vi "Typhon_Software-RevE.vi"() -> ()   [LabVIEW 2020]
uses:
  <vilib>/DAQmx/write.llb/DAQmx Write (Digital 1D Bool 1Chan 1Samp).vi
  <vilib>/DAQmx/read.llb/DAQmx Read (Analog 1D DBL NChan 1Samp).vi
  <vilib>/Utility/file.llb/Write Delimited Spreadsheet (string).vi
  <vilib>/DAQmx/create/channels.llb/DAQmx Create Channel (AI-Voltage-Basic).vi
  <vilib>/DAQmx/configure/timing.llb/DAQmx Timing (Sample Clock).vi
  <vilib>/DAQmx/miscellaneous.llb/DAQmx Fill In Error Info.vi
  <vilib>/Utility/file.llb/Write Delimited Spreadsheet (DBL).vi
  <vilib>/DAQmx/create/channels.llb/DAQmx Create Channel (DO-Digital Output).vi
panel:
  out "Temp 3":dbl(graph)
  out "Temp 2":dbl(graph)
  out "Load mV":dbl(graph)
  out "time":timestamp
  in  "stop":bool
  out "Temp 1":dbl(graph)
  out "Thrust":dbl
  out "Temp 3":dbl
  out "Temp 2":dbl
  out "Temp 1":dbl
  in  "Force":path
  in  "Temperature":path
  out "E-Match":bool
  out "N2-CH4":bool
  out "N2-GOX":bool
  out "CH4  Isolation":bool
  out "CH4  Upper":bool
  out "GOX Isolation":bool
  out "GOX Upper":bool
  out "State":i32
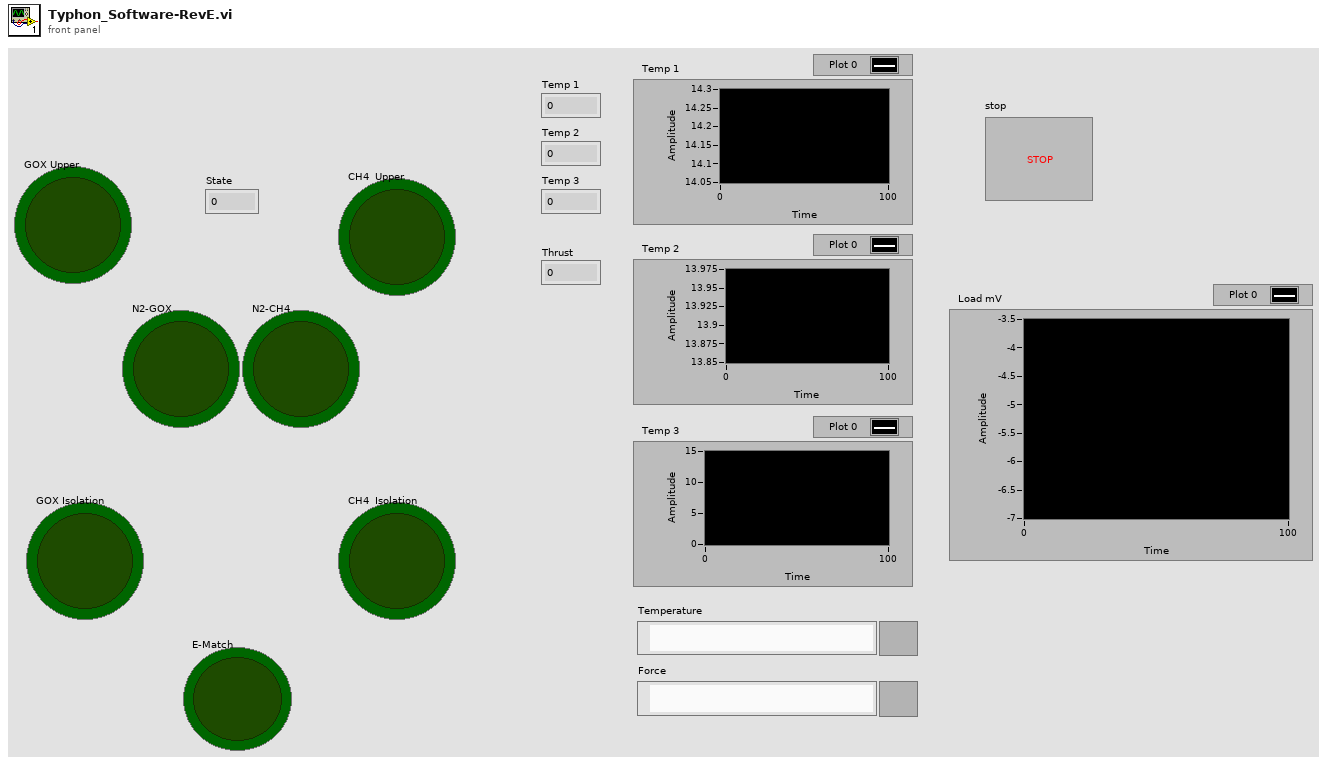
[diagram p1: front panel]
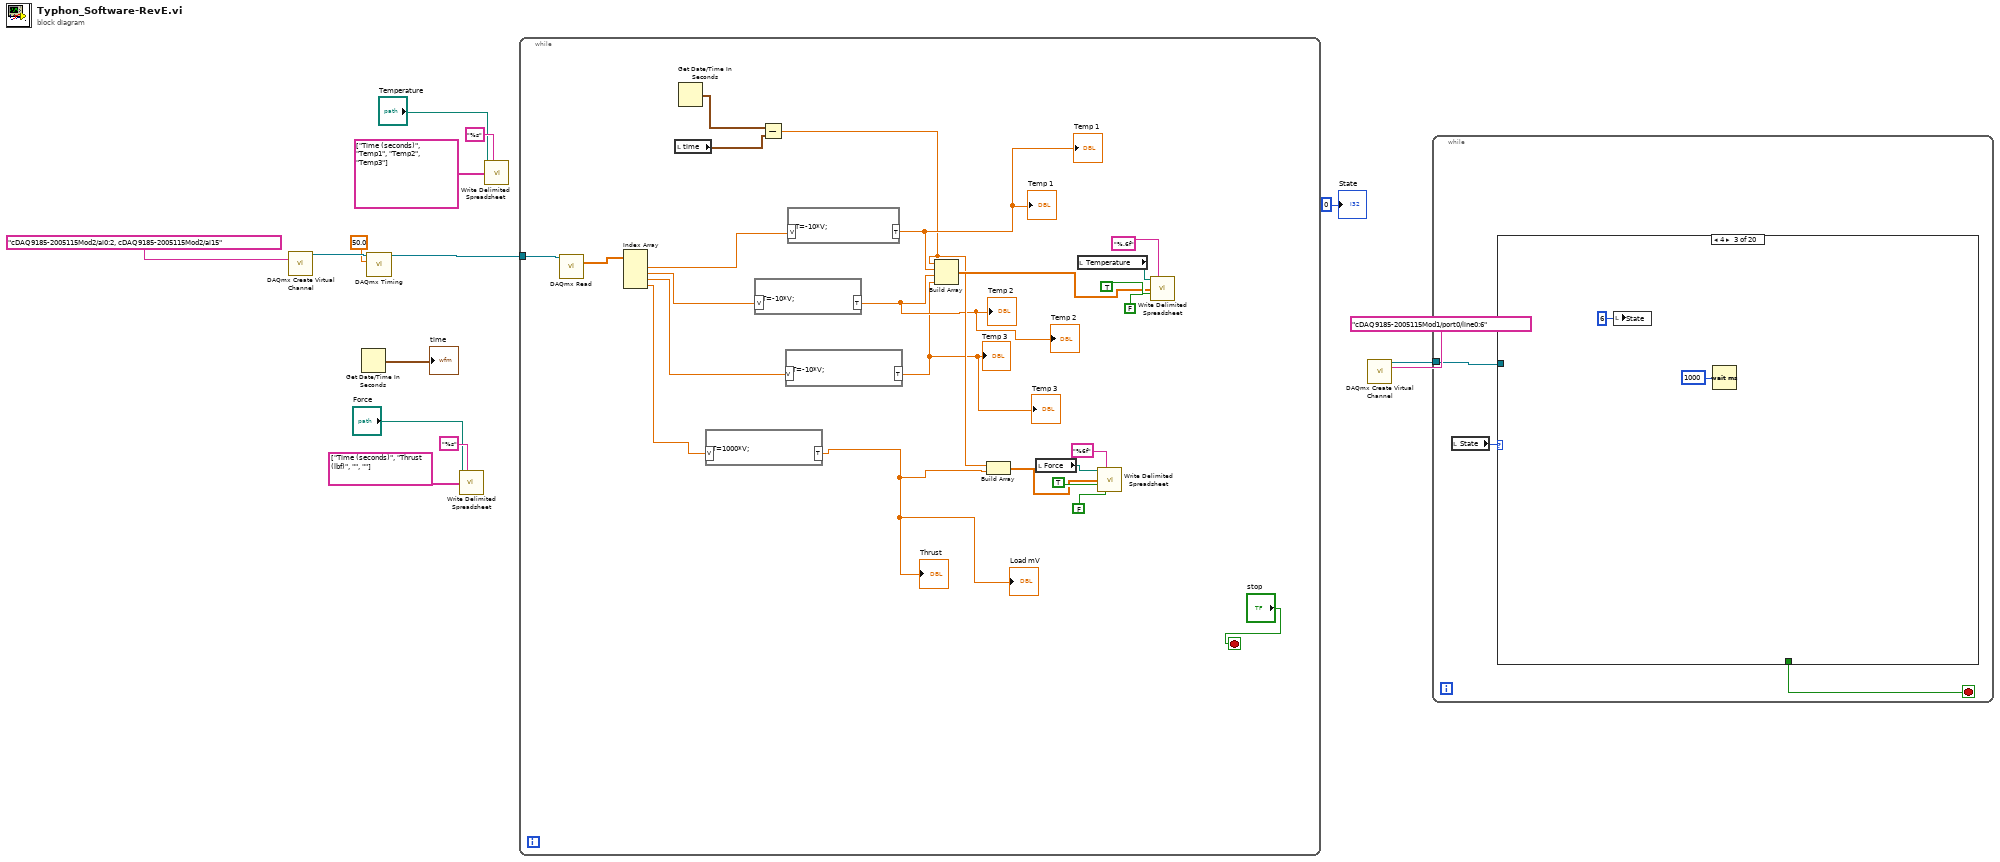
[diagram p0: block diagram]
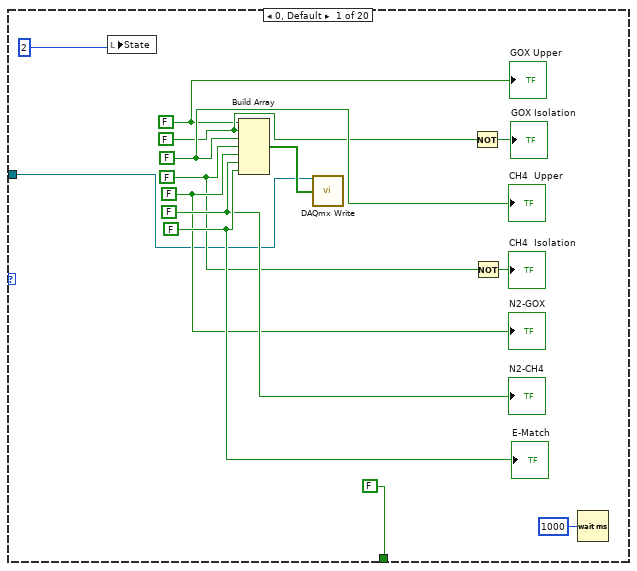
[diagram p2: hidden frame]
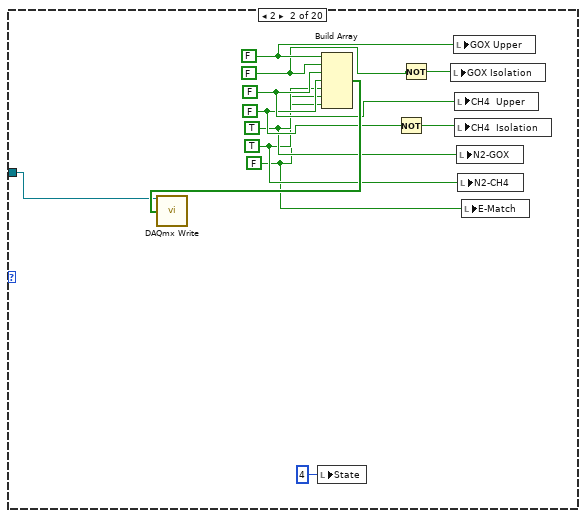
[diagram p3: hidden frame]
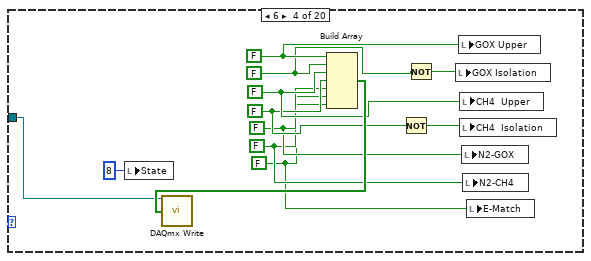
[diagram p4: hidden frame]
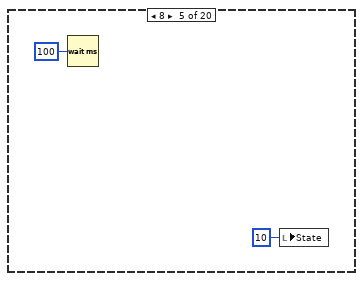
[diagram p5: hidden frame]
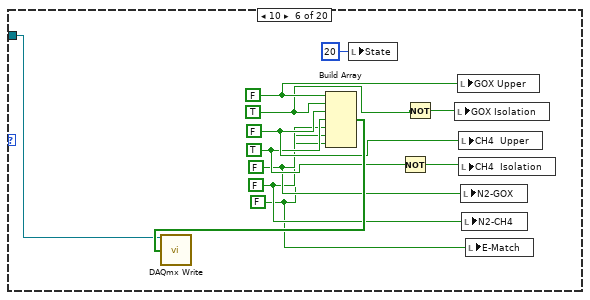
[diagram p6: hidden frame]
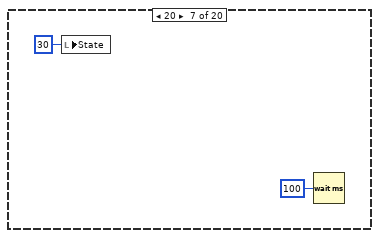
[diagram p7: hidden frame]
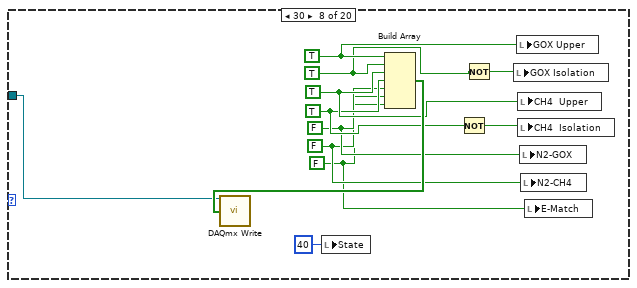
[diagram p8: hidden frame]
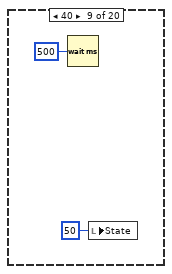
[diagram p9: hidden frame]
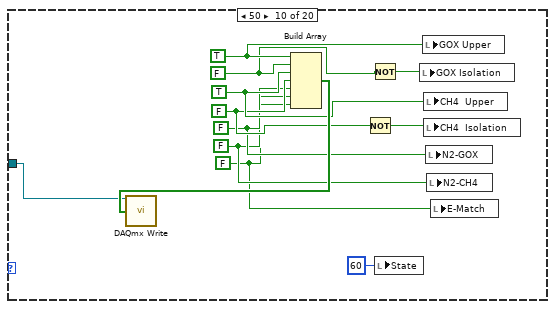
[diagram p10: hidden frame]
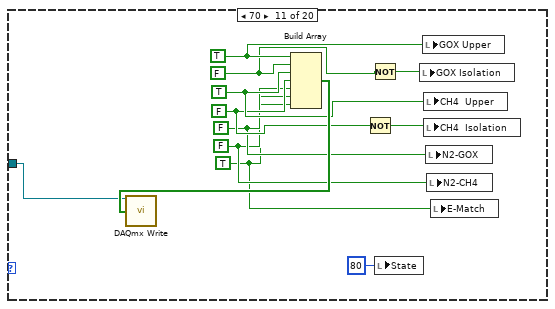
[diagram p11: hidden frame]
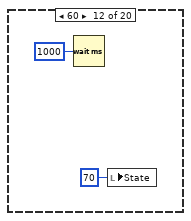
[diagram p12: hidden frame]
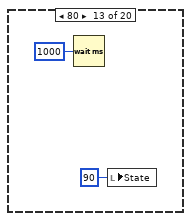
[diagram p13: hidden frame]
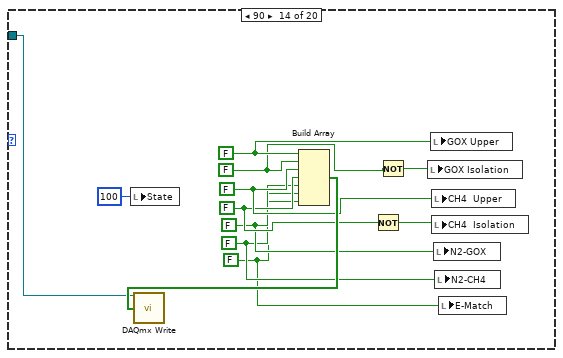
[diagram p14: hidden frame]
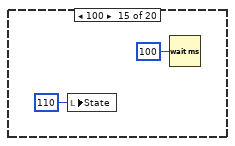
[diagram p15: hidden frame]
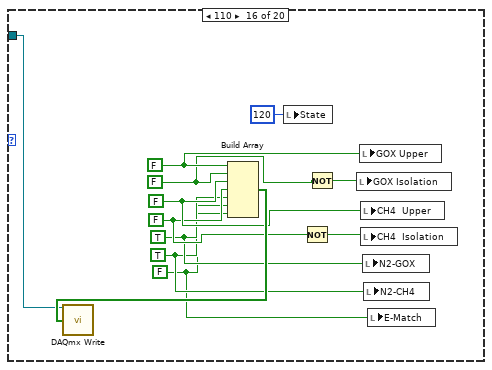
[diagram p16: hidden frame]
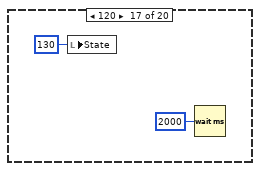
[diagram p17: hidden frame]
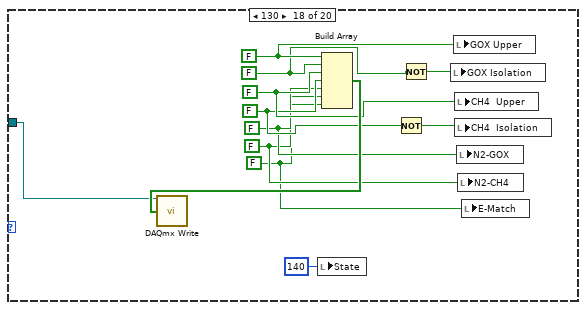
[diagram p18: hidden frame]
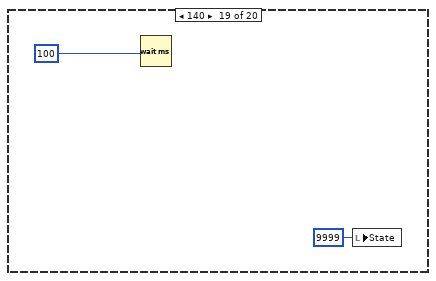
[diagram p19: hidden frame]
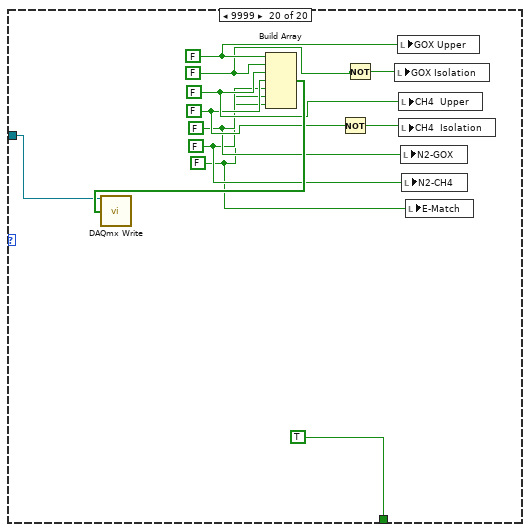
[diagram p20: hidden frame]
diagram:
  n1 = call-poly <vilib>:"DAQmx Create Virtual Channel.vi"("physical channels"=tag "cDAQ9185-2005115Mod2/ai0:2, cDAQ9185-2005115Mod2/ai15") -> ("task out"=w10:refnum<k21>)  [unwired: 13 in, 1 out]
  n2 = Get Date/Time In Seconds() -> (seconds since 1Jan1904=→"time":timestamp)
  n3 = call-poly <vilib>:"DAQmx Timing.vi"("task/channels in"=w10, "rate"=50.0) -> ("task out"=w7:refnum<k21>)  [unwired: 12 in, 1 out]
  n4 = call-poly <vilib>:"Write Delimited Spreadsheet.vi"("file path (dialog if empty)"="Force", "format (%s)"="%s" ("format (%.3f)"), "1D data"=string[] ["Time (seconds)", "Thrust (lbf)", "", ""]) -> ()  [unwired: 11 in, 2 out]
  n5 = call-poly <vilib>:"Write Delimited Spreadsheet.vi"("file path (dialog if empty)"="Temperature", "format (%s)"="%s" ("format (%.3f)"), "1D data"=string[] ["Time (seconds)", "Temp1", "Temp2", "Temp3"]) -> ()  [unwired: 11 in, 2 out]
  n6 = while {
    tunnel: w7 -> [w33]
    stop <- "stop" stop-if-true
    n7 = call-poly <vilib>:"DAQmx Read.vi"("task/channels in"=w33) -> ("data"=w34:dbl[])  [unwired: 12 in, 2 out]
    n8 = Index Array(array=w34) -> (element #1=w29:dbl, element #2=w28:dbl, element #3=w27:dbl, element #4=w18:dbl)  [unwired: 4 in]
    n9 = local read "time"() -> (w20:timestamp)
    n10 = Get Date/Time In Seconds() -> (seconds since 1Jan1904=w21:timestamp)
    n11 = formula code="T=1000*V;"("V"=w18) -> ("T"=w17:dbl)
    "Thrust" <- w17
    "Load mV" <- w17
    n12 = formula code="T=-10*V;"("V"=w28) -> ("T"=w16:dbl)
    "Temp 2" <- w16
    "Temp 2" <- w16
    n13 = Subtract(x=w21, y=w20) -> (x-y=w22:dbl)
    n14 = formula code="T=-10*V;"("V"=w27) -> ("T"=w15:dbl)
    "Temp 3" <- w15
    "Temp 3" <- w15
    n15 = formula code="T=-10*V;"("V"=w29) -> ("T"=w26:dbl)
    "Temp 1" <- w26
    "Temp 1" <- w26
    n16 = Build Array(w22, w26, w16, w15) -> (w24:dbl[])
    n17 = Build Array(w22, w17) -> (w19:dbl[])
    n18 = local read "Force"() -> (w30:path)
    n19 = local read "Temperature"() -> (w35:path)
    n20 = call-poly <vilib>:"Write Delimited Spreadsheet.vi"("file path (dialog if empty)"=w30, "format (%.3f)"="%6f", "1D data"=w19, "append to file? (new file:F)"=TRUE, "transpose? (no:F)"=FALSE) -> ()  [unwired: 9 in, 2 out]
    n21 = call-poly <vilib>:"Write Delimited Spreadsheet.vi"("file path (dialog if empty)"=w35, "format (%.3f)"="%.6f", "1D data"=w24, "append to file? (new file:F)"=TRUE, "transpose? (no:F)"=FALSE) -> ()  [unwired: 9 in, 2 out]
  }
  n22 = call-poly <vilib>:"DAQmx Create Virtual Channel.vi"("lines"=tag "cDAQ9185-2005115Mod1/port0/line0:6") -> ("task out"=w2:refnum<k21>)  [unwired: 13 in, 1 out]
  n23 = while {
    tunnel: w2 -> [w40]
    stop <- w39 stop-if-true
    n24 = local read "State"() -> (w41:i32)
    n25 = case shown="4" w41 {
      tunnel: [FALSE _ _ _ _ _ _ _ _ _ _ _ _ _ _ _ _ _ _ TRUE] -> w39
      tunnel: w40 -> [w42 w56 _ w70 _ w84 _ w98 _ w112 w124 _ _ w140 _ w154 _ w168 _ w182]
      frame 0, Default {
        w49 = FALSE ("element")
        w48 = FALSE ("element")
        w47 = FALSE ("element")
        w46 = FALSE ("element")
        w45 = FALSE ("element")
        w44 = FALSE
        w43 = FALSE
        n26 = local write "State"(2 ("State")) -> ()
        n27 = Build Array(w43, w44, w45, w46, w47, w48, w49) -> (w50:bool[])
        n28 = call-poly <vilib>:"DAQmx Write.vi"("task/channels in"=w42, "data"=w50) -> ()  [unwired: 11 in, 3 out]
        n29 = Not(x=w44) -> (.not. x?=→"GOX Isolation":bool)
        n30 = Not(x=w46) -> (.not. x?=→"CH4  Isolation":bool)
        n31 = Wait (ms)(milliseconds to wait=u32 1000) -> ()  [unwired: 1 out]
        "GOX Upper" <- w43
        "CH4  Upper" <- w45
        "N2-GOX" <- w47
        "N2-CH4" <- w48
        "E-Match" <- w49
      }
      frame 2 {
        w57 = FALSE ("element")
        w58 = TRUE ("element")
        w59 = TRUE ("element")
        w60 = FALSE ("element")
        w61 = FALSE ("element")
        w62 = FALSE
        w63 = FALSE
        n32 = local write "State"(4 ("State")) -> ()
        n33 = Build Array(w63, w62, w61, w60, w59, w58, w57) -> (w66:bool[])
        n34 = call-poly <vilib>:"DAQmx Write.vi"("task/channels in"=w56, "data"=w66) -> ()  [unwired: 11 in, 3 out]
        n35 = Not(x=w60) -> (.not. x?=w65:bool)
        n36 = Not(x=w62) -> (.not. x?=w64:bool)
        n37 = local write "GOX Isolation"(w64) -> ()
        n38 = local write "GOX Upper"(w63) -> ()
        n39 = local write "CH4  Upper"(w61) -> ()
        n40 = local write "CH4  Isolation"(w65) -> ()
        n41 = local write "N2-GOX"(w59) -> ()
        n42 = local write "N2-CH4"(w58) -> ()
        n43 = local write "E-Match"(w57) -> ()
      }
      frame 4 {
        n44 = local write "State"(6 ("State")) -> ()
        n45 = Wait (ms)(milliseconds to wait=u32 1000) -> ()  [unwired: 1 out]
      }
      frame 6 {
        w71 = FALSE ("element")
        w72 = FALSE ("element")
        w73 = FALSE ("element")
        w74 = FALSE ("element")
        w75 = FALSE ("element")
        w76 = FALSE
        w77 = FALSE
        n46 = local write "State"(8 ("State")) -> ()
        n47 = Build Array(w77, w76, w75, w74, w73, w72, w71) -> (w80:bool[])
        n48 = call-poly <vilib>:"DAQmx Write.vi"("task/channels in"=w70, "data"=w80) -> ()  [unwired: 11 in, 3 out]
        n49 = Not(x=w74) -> (.not. x?=w79:bool)
        n50 = Not(x=w76) -> (.not. x?=w78:bool)
        n51 = local write "GOX Isolation"(w78) -> ()
        n52 = local write "GOX Upper"(w77) -> ()
        n53 = local write "CH4  Upper"(w75) -> ()
        n54 = local write "CH4  Isolation"(w79) -> ()
        n55 = local write "N2-GOX"(w73) -> ()
        n56 = local write "N2-CH4"(w72) -> ()
        n57 = local write "E-Match"(w71) -> ()
      }
      frame 8 {
        n58 = Wait (ms)(milliseconds to wait=u32 100) -> ()  [unwired: 1 out]
        n59 = local write "State"(10 ("State")) -> ()
      }
      frame 10 {
        w85 = FALSE ("element")
        w86 = FALSE ("element")
        w87 = FALSE ("element")
        w88 = TRUE ("element")
        w89 = FALSE ("element")
        w90 = TRUE
        w91 = FALSE
        n60 = Build Array(w91, w90, w89, w88, w87, w86, w85) -> (w94:bool[])
        n61 = call-poly <vilib>:"DAQmx Write.vi"("task/channels in"=w84, "data"=w94) -> ()  [unwired: 11 in, 3 out]
        n62 = local write "State"(20 ("State")) -> ()
        n63 = Not(x=w88) -> (.not. x?=w93:bool)
        n64 = Not(x=w90) -> (.not. x?=w92:bool)
        n65 = local write "GOX Isolation"(w92) -> ()
        n66 = local write "GOX Upper"(w91) -> ()
        n67 = local write "CH4  Upper"(w89) -> ()
        n68 = local write "CH4  Isolation"(w93) -> ()
        n69 = local write "N2-GOX"(w87) -> ()
        n70 = local write "N2-CH4"(w86) -> ()
        n71 = local write "E-Match"(w85) -> ()
      }
      frame 20 {
        n72 = local write "State"(30 ("State")) -> ()
        n73 = Wait (ms)(milliseconds to wait=u32 100) -> ()  [unwired: 1 out]
      }
      frame 30 {
        w99 = FALSE ("element")
        w100 = FALSE ("element")
        w101 = FALSE ("element")
        w102 = TRUE ("element")
        w103 = TRUE ("element")
        w104 = TRUE
        w105 = TRUE
        n74 = local write "State"(40 ("State")) -> ()
        n75 = Build Array(w105, w104, w103, w102, w101, w100, w99) -> (w108:bool[])
        n76 = call-poly <vilib>:"DAQmx Write.vi"("task/channels in"=w98, "data"=w108) -> ()  [unwired: 11 in, 3 out]
        n77 = Not(x=w102) -> (.not. x?=w107:bool)
        n78 = Not(x=w104) -> (.not. x?=w106:bool)
        n79 = local write "GOX Isolation"(w106) -> ()
        n80 = local write "GOX Upper"(w105) -> ()
        n81 = local write "CH4  Upper"(w103) -> ()
        n82 = local write "CH4  Isolation"(w107) -> ()
        n83 = local write "N2-GOX"(w101) -> ()
        n84 = local write "N2-CH4"(w100) -> ()
        n85 = local write "E-Match"(w99) -> ()
      }
      frame 40 {
        n86 = Wait (ms)(milliseconds to wait=u32 500) -> ()  [unwired: 1 out]
        n87 = local write "State"(50 ("State")) -> ()
      }
      frame 50 {
        w113 = FALSE ("element")
        w114 = FALSE ("element")
        w115 = FALSE ("element")
        w116 = FALSE ("element")
        w117 = TRUE ("element")
        w118 = FALSE
        w119 = TRUE
        n88 = Build Array(w119, w118, w117, w116, w115, w114, w113) -> (w122:bool[])
        n89 = call-poly <vilib>:"DAQmx Write.vi"("task/channels in"=w112, "data"=w122) -> ()  [unwired: 11 in, 3 out]
        n90 = Not(x=w116) -> (.not. x?=w121:bool)
        n91 = Not(x=w118) -> (.not. x?=w120:bool)
        n92 = local write "State"(60 ("State")) -> ()
        n93 = local write "GOX Isolation"(w120) -> ()
        n94 = local write "GOX Upper"(w119) -> ()
        n95 = local write "CH4  Upper"(w117) -> ()
        n96 = local write "CH4  Isolation"(w121) -> ()
        n97 = local write "N2-GOX"(w115) -> ()
        n98 = local write "N2-CH4"(w114) -> ()
        n99 = local write "E-Match"(w113) -> ()
      }
      frame 70 {
        w125 = TRUE ("element")
        w126 = FALSE ("element")
        w127 = FALSE ("element")
        w128 = FALSE ("element")
        w129 = TRUE ("element")
        w130 = FALSE
        w131 = TRUE
        n100 = Build Array(w131, w130, w129, w128, w127, w126, w125) -> (w134:bool[])
        n101 = call-poly <vilib>:"DAQmx Write.vi"("task/channels in"=w124, "data"=w134) -> ()  [unwired: 11 in, 3 out]
        n102 = Not(x=w128) -> (.not. x?=w133:bool)
        n103 = Not(x=w130) -> (.not. x?=w132:bool)
        n104 = local write "State"(80 ("State")) -> ()
        n105 = local write "GOX Isolation"(w132) -> ()
        n106 = local write "GOX Upper"(w131) -> ()
        n107 = local write "CH4  Upper"(w129) -> ()
        n108 = local write "CH4  Isolation"(w133) -> ()
        n109 = local write "N2-GOX"(w127) -> ()
        n110 = local write "N2-CH4"(w126) -> ()
        n111 = local write "E-Match"(w125) -> ()
      }
      frame 60 {
        n112 = Wait (ms)(milliseconds to wait=u32 1000) -> ()  [unwired: 1 out]
        n113 = local write "State"(70 ("State")) -> ()
      }
      frame 80 {
        n114 = Wait (ms)(milliseconds to wait=u32 1000) -> ()  [unwired: 1 out]
        n115 = local write "State"(90 ("State")) -> ()
      }
      frame 90 {
        w141 = FALSE ("element")
        w142 = FALSE ("element")
        w143 = FALSE ("element")
        w144 = FALSE ("element")
        w145 = FALSE ("element")
        w146 = FALSE
        w147 = FALSE
        n116 = local write "State"(100 ("State")) -> ()
        n117 = Build Array(w147, w146, w145, w144, w143, w142, w141) -> (w150:bool[])
        n118 = call-poly <vilib>:"DAQmx Write.vi"("task/channels in"=w140, "data"=w150) -> ()  [unwired: 11 in, 3 out]
        n119 = Not(x=w144) -> (.not. x?=w149:bool)
        n120 = Not(x=w146) -> (.not. x?=w148:bool)
        n121 = local write "GOX Isolation"(w148) -> ()
        n122 = local write "GOX Upper"(w147) -> ()
        n123 = local write "CH4  Upper"(w145) -> ()
        n124 = local write "CH4  Isolation"(w149) -> ()
        n125 = local write "N2-GOX"(w143) -> ()
        n126 = local write "N2-CH4"(w142) -> ()
        n127 = local write "E-Match"(w141) -> ()
      }
      frame 100 {
        n128 = local write "State"(110 ("State")) -> ()
        n129 = Wait (ms)(milliseconds to wait=u32 100) -> ()  [unwired: 1 out]
      }
      frame 110 {
        w155 = FALSE ("element")
        w156 = TRUE ("element")
        w157 = TRUE ("element")
        w158 = FALSE ("element")
        w159 = FALSE ("element")
        w160 = FALSE
        w161 = FALSE
        n130 = Build Array(w161, w160, w159, w158, w157, w156, w155) -> (w164:bool[])
        n131 = call-poly <vilib>:"DAQmx Write.vi"("task/channels in"=w154, "data"=w164) -> ()  [unwired: 11 in, 3 out]
        n132 = local write "State"(120 ("State")) -> ()
        n133 = Not(x=w158) -> (.not. x?=w163:bool)
        n134 = Not(x=w160) -> (.not. x?=w162:bool)
        n135 = local write "GOX Isolation"(w162) -> ()
        n136 = local write "GOX Upper"(w161) -> ()
        n137 = local write "CH4  Upper"(w159) -> ()
        n138 = local write "CH4  Isolation"(w163) -> ()
        n139 = local write "N2-GOX"(w157) -> ()
        n140 = local write "N2-CH4"(w156) -> ()
        n141 = local write "E-Match"(w155) -> ()
      }
      frame 120 {
        n142 = local write "State"(130 ("State")) -> ()
        n143 = Wait (ms)(milliseconds to wait=u32 2000) -> ()  [unwired: 1 out]
      }
      frame 130 {
        w169 = FALSE ("element")
        w170 = FALSE ("element")
        w171 = FALSE ("element")
        w172 = FALSE ("element")
        w173 = FALSE ("element")
        w174 = FALSE
        w175 = FALSE
        n144 = local write "State"(140 ("State")) -> ()
        n145 = Build Array(w175, w174, w173, w172, w171, w170, w169) -> (w178:bool[])
        n146 = call-poly <vilib>:"DAQmx Write.vi"("task/channels in"=w168, "data"=w178) -> ()  [unwired: 11 in, 3 out]
        n147 = Not(x=w172) -> (.not. x?=w177:bool)
        n148 = Not(x=w174) -> (.not. x?=w176:bool)
        n149 = local write "GOX Isolation"(w176) -> ()
        n150 = local write "GOX Upper"(w175) -> ()
        n151 = local write "CH4  Upper"(w173) -> ()
        n152 = local write "CH4  Isolation"(w177) -> ()
        n153 = local write "N2-GOX"(w171) -> ()
        n154 = local write "N2-CH4"(w170) -> ()
        n155 = local write "E-Match"(w169) -> ()
      }
      frame 140 {
        n156 = Wait (ms)(milliseconds to wait=u32 100) -> ()  [unwired: 1 out]
        n157 = local write "State"(9999 ("State")) -> ()
      }
      frame 9999 {
        w183 = FALSE ("element")
        w184 = FALSE ("element")
        w185 = FALSE ("element")
        w186 = FALSE ("element")
        w187 = FALSE ("element")
        w188 = FALSE
        w189 = FALSE
        n158 = Build Array(w189, w188, w187, w186, w185, w184, w183) -> (w192:bool[])
        n159 = call-poly <vilib>:"DAQmx Write.vi"("task/channels in"=w182, "data"=w192) -> ()  [unwired: 11 in, 3 out]
        n160 = Not(x=w186) -> (.not. x?=w191:bool)
        n161 = Not(x=w188) -> (.not. x?=w190:bool)
        n162 = local write "GOX Isolation"(w190) -> ()
        n163 = local write "GOX Upper"(w189) -> ()
        n164 = local write "CH4  Upper"(w187) -> ()
        n165 = local write "CH4  Isolation"(w191) -> ()
        n166 = local write "N2-GOX"(w185) -> ()
        n167 = local write "N2-CH4"(w184) -> ()
        n168 = local write "E-Match"(w183) -> ()
      }
    }
  }
  "State" <- 0 ("State")
